vi "sub_temp_data_maping.vi"(11 "temp_data":dbl[][](array[numeric])) -> (1 "mean":dbl caption="temp mean" format="%0.2f", 2 "intensity":dbl[][](array[numeric]), 3 "mapping_temp":dbl[][](array[numeric]))   [LabVIEW 2013]
uses:
  <vilib>/Analysis/baseanly.llb/Mean (DBL).vi
  <vilib>/Analysis/NI_AALBase.lvlib
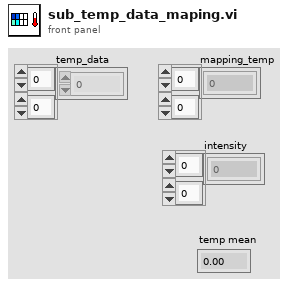
[diagram p1: front panel]
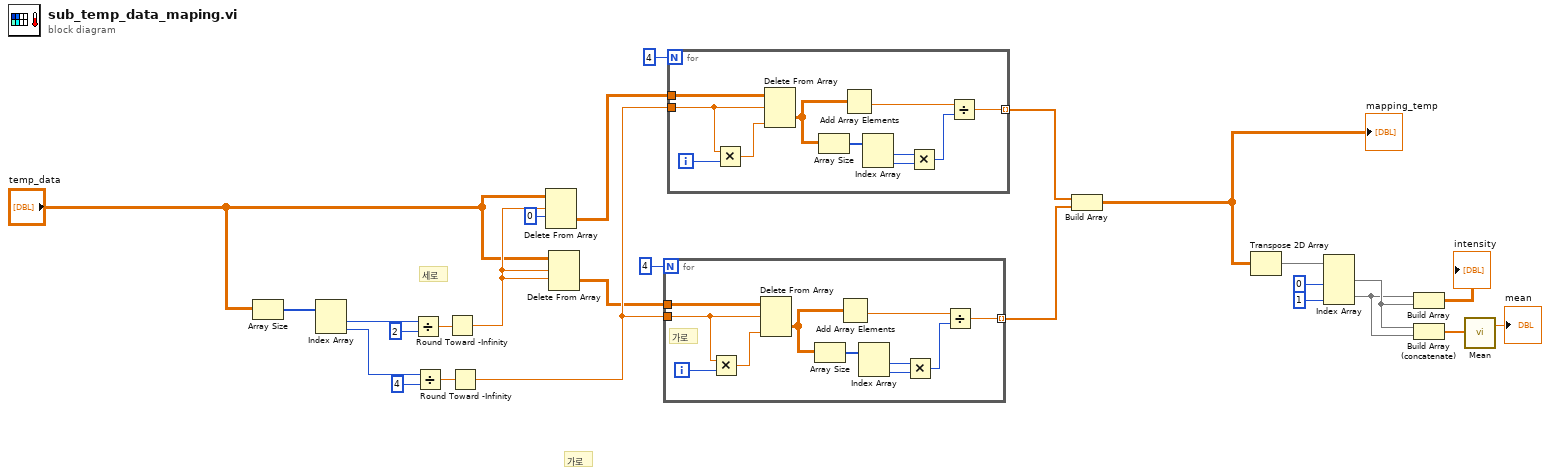
[diagram p0: block diagram]
diagram:
  # "가로"
  # "세로"
  n1 = Array Size(array="temp_data") -> (size(s)=w18:i32[])
  n2 = Index Array(array=w18) -> (element #1=w23:i32, element #2=w24:i32)  [unwired: 2 in]
  n3 = Divide(x=w23, y=2) -> (x/y=w20:dbl)
  n4 = Divide(x=w24, y=4) -> (x/y=w19:dbl)
  n5 = Round Toward -Infinity(1:w20) -> (0:w26:dbl)
  n6 = Round Toward -Infinity(1:w19) -> (0:w25:dbl)
  n7 = Delete From Array(array="temp_data", length=w26, index (row)=0 ("인덱스 (행)")) -> (deleted portion=w12:dbl[][])  [unwired: 1 in, 1 out]
  n8 = Delete From Array(array="temp_data", length=w26, index (row)=w26) -> (deleted portion=w15:dbl[][])  [unwired: 1 in, 1 out]
  n9 = for {
    N: 4 -> [_]
    tunnel: w25 -> [w35]
    tunnel: w15 -> [w37]
    tunnel: [w29] -> w16 mode=indexing
    i -> [w36]
    # "가로"
    n10 = Multiply(x=w35, y=w36) -> (x*y=w34:dbl)
    n11 = Delete From Array(array=w37, length=w35, index (col)=w34) -> (deleted portion=w33:dbl[][])  [unwired: 1 in, 1 out]
    n12 = Array Size(array=w33) -> (size(s)=w32:i32[])
    n13 = Add Array Elements(numeric array=w33) -> (sum=w28:dbl)
    n14 = Index Array(array=w32) -> (element #1=w31:i32, element #2=w30:i32)  [unwired: 2 in]
    n15 = Multiply(x=w31, y=w30) -> (x*y=w27:i32)
    n16 = Divide(x=w28, y=w27) -> (x/y=w29:dbl)
  }
  n17 = for {
    N: 4 -> [_]
    tunnel: w25 -> [w46]
    tunnel: w12 -> [w48]
    tunnel: [w40] -> w13 mode=indexing
    i -> [w47]
    n18 = Multiply(x=w46, y=w47) -> (x*y=w45:dbl)
    n19 = Delete From Array(array=w48, length=w46, index (col)=w45) -> (deleted portion=w44:dbl[][])  [unwired: 1 in, 1 out]
    n20 = Array Size(array=w44) -> (size(s)=w43:i32[])
    n21 = Add Array Elements(numeric array=w44) -> (sum=w39:dbl)
    n22 = Index Array(array=w43) -> (element #1=w42:i32, element #2=w41:i32)  [unwired: 2 in]
    n23 = Multiply(x=w42, y=w41) -> (x*y=w38:i32)
    n24 = Divide(x=w39, y=w38) -> (x/y=w40:dbl)
  }
  n25 = Build Array(w13, w16) -> (w1:dbl[][])
  "mapping_temp" <- w1
  n26 = Transpose 2D Array(2D array=w1) -> (transposed array=w7:dbl[][])
  n27 = Index Array(array=w7, index (col) #1=0 ("비활성화된 인덱스 (열)"), index (col) #2=1 ("비활성화된 인덱스 (열)")) -> (element #1=w6:dbl[], element #2=w5:dbl[])  [unwired: 2 in]
  n28 = Build Array(w5, w6) -> (→"intensity":dbl[][])
  n29 = Build Array (concatenate)(w6, w5) -> (w4:dbl[])
  n30 = call-poly <vilib>:"Mean.vi"("X"=w4) -> ("mean"=→"mean":dbl)  [unwired: 1 out]
